vi "readMotorEnc.vi"(6 "Reset Counter":bool, 7 "Reverse ENC?":bool, 8 "error in (no error)":errorcluster) -> (0 "error out":errorcluster, 2 "MotorEncoder (deg)":dbl)   [LabVIEW 2019, in "SJCube_KNRm.lvlib"]
uses:
  SJCube_KNRm.lvlib
  KNRm_ReMi_OS5.lvlibp/KNRm_ReMi_Toolkit/IO/LowLevel/IO_Channel_Motor.ctl
  KNRm_ReMi_OS5.lvlibp
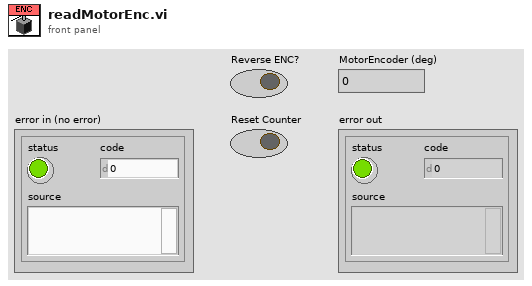
[diagram p1: front panel]
types:
  T1 = typedef "KNRm_ReMi_OS5.lvlibp/IO_Channel_Motor.ctl" = enum16{"M1", "M2", "M3", "M4"}
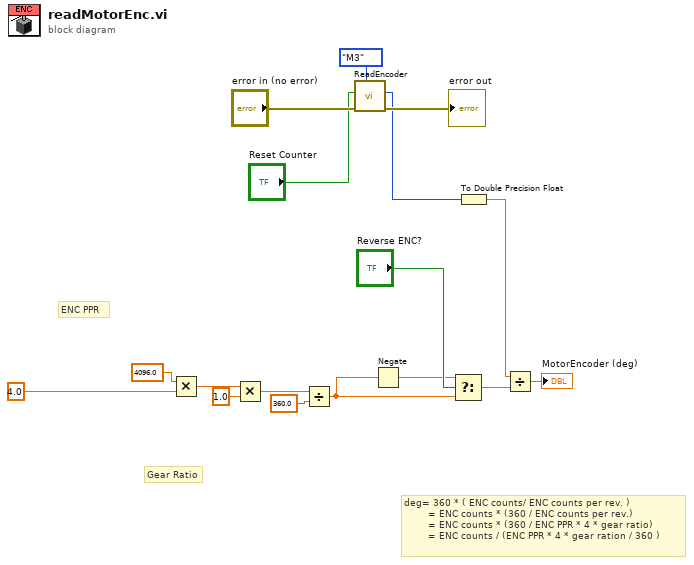
[diagram p0: block diagram]
diagram:
  # "Gear Ratio"
  # "ENC PPR"
  # "deg= 360 * ( ENC counts/ ENC counts per rev. )\n        = ENC counts * (360 / ENC counts per rev.)\n        = ENC counts * (360 / ENC PPR * 4 * gear ratio)\n        = ENC counts / (ENC PPR * 4 * gear ration / 360 )"
  n1 = Multiply(x=4096.0 ("y"), y=4.0) -> (x*y=w11:dbl)
  n2 = Multiply(x=w11, y=1.0) -> (x*y=w9:dbl)
  n3 = Divide(x=w9, y=360.0) -> (x/y=w6:dbl)
  n4 = call "ReadEncoder.vi"("Channel"=IO_Channel_Motor."M3", "error in"="error in (no error)", "Reset"="Reset Counter") -> ("error out"=→"error out":errorcluster, "ENC (count)"=w1:i32)  [unwired: 7 in]
  n5 = Negate(x=w6) -> (-x=w7:dbl)
  n6 = Select(t=w7, s="Reverse ENC?", f=w6) -> (s? t:f=w14:dbl)
  n7 = To Double Precision Float(number=w1) -> (double precision float=w16:dbl)
  n8 = Divide(x=w16, y=w14) -> (x/y=→"MotorEncoder (deg)":dbl)
